vi "test Check Main Properties Changes.vi"(8 "error in":errorcluster, 11 "TestCase in":refnum<class "AIM ARINC 664 EncodeDecode.lvclass">) -> (0 "error out":errorcluster, 3 "TestCase out":refnum<class "AIM ARINC 664 EncodeDecode.lvclass">)   [LabVIEW 2020, in "AIM ARINC 664 EncodeDecode.lvclass"]
uses:
  AIM ARINC 664 EncodeDecode.lvclass
  C:/Program Files (x86)/National Instruments/LabVIEW 2020/vi.lib/NI/VeriStand Custom Device Testing Tools/VeriStandScriptingTestCase/VeriStandScriptingTestCase.lvclass
  Import/_typedefs/session_tx_generic.ctl
  Import/_typedefs/tx_generic_setup.ctl
  Import/_typedefs/frame_tx_generic.ctl
  Import/_typedefs/frame_tx_generic_seqNumberInit.ctl
  Import/_typedefs/frame_tx_generic_seqNumberOffset.ctl
  Import/_typedefs/frame_parameter.ctl
  Import/_typedefs/frame_parameter_definition.ctl
  <vilib>/NI/NI VeriStand Encoding and Decoding/Encoding.ctl
  Import/_typedefs/session_rx_monitor.ctl
  Import/_typedefs/board_setup.ctl
  <vilib>/NI/VeriStand Custom Device Testing Tools/VeriStandScriptingTestCase/VeriStandScriptingTestCase.lvclass/VeriStandScriptingTestCase.ctl
  <vilib>/NI/VeriStand Custom Device Testing Tools/VeriStandScriptingTestCase/Read Target.vi
  NationalInstruments.VeriStand.SystemDefinitionAPI
  <vilib>/addons/_JKI Toolkits/VI Tester/TestCase.llb/TestCase.lvclass
  Scripting/AIM ARINC 664 Scripting.lvlib
  Import/AIM ARINC 664 Import.lvlib
  <vilib>/NI/NI VeriStand Encoding and Decoding/Encoding and Decoding.lvlib
  C:/Program Files (x86)/National Instruments/LabVIEW 2020/vi.lib/addons/_JKI Toolkits/VI Tester/TestCase.llb/TestCase.lvclass
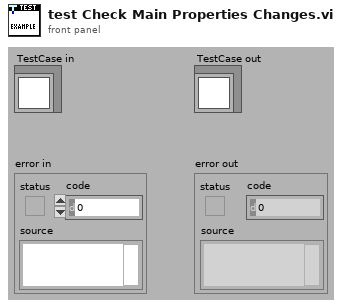
[diagram p1: front panel]
types:
  T1 = typedef "AIM ARINC 664 Import.lvlib/session_rx_monitor.ctl" = cluster{"DefaultCronoMode":u32, "GlbMonBufferSizeIn":u32, "CaptureMode":u32, "MaxFileSizeMB":u32, "Strobe":u32, "TriggerPosition":u32}
  T2 = typedef "AIM ARINC 664 Import.lvlib/session_tx_generic.ctl" = cluster{"tx_generic_setup":T3, "Frame Headers":T4[]}
  T3 = typedef "AIM ARINC 664 Import.lvlib/tx_generic_setup.ctl" = cluster{"QueueSizeIn":u32, "Count":i32, "StartMode":i32}
  T4 = typedef "AIM ARINC 664 Import.lvlib/frame_tx_generic.ctl" = cluster{"FrameID":string, "PayloadID":string, "Frame header":cluster{"FrameStartMode":i32, "InterFrameGap":i32, "PacketGroupWaitTime":i32, "NetSelect":u32, "PayloadBufferMode":i32, "PayloadGenerationMode":i32, "PhysErrorInjection":i32, "PreambleCount":i32, "SequenceNumberInit":T5, "SequenceNumberOffset":T6, "Skew":i32}, "Parameters":T7[]}
  T5 = typedef "AIM ARINC 664 Import.lvlib/frame_tx_generic_seqNumberInit.ctl" = i32
  T6 = typedef "AIM ARINC 664 Import.lvlib/frame_tx_generic_seqNumberOffset.ctl" = i32
  T7 = typedef "AIM ARINC 664 Import.lvlib/frame_parameter.ctl" = cluster{"name":string, "default value":dbl, "unit":string, "Parameter":T8}
  T8 = typedef "AIM ARINC 664 Import.lvlib/frame_parameter_definition.ctl" = cluster{"start index":i32, "size":i32, "encoding":T9, "signed":bool, "scale multiplier":dbl, "scale offset":dbl}
  T9 = typedef "Encoding and Decoding.lvlib/Encoding.ctl" = enum16{"BNR", "BCD", "Discrete"}
  T10 = typedef "AIM ARINC 664 Import.lvlib/board_setup.ctl" = cluster{"boardId":u32, "portSpeed":u32, "portConfig":u32}
  T11 = typedef "Custom Device API.lvlib/Custom Device Item Ref.ctl" = u64
  T12 = typedef "AIM ARINC 664 Import.lvlib/port_setup.ctl" = cluster{"port Id":u32, "redundant":bool}
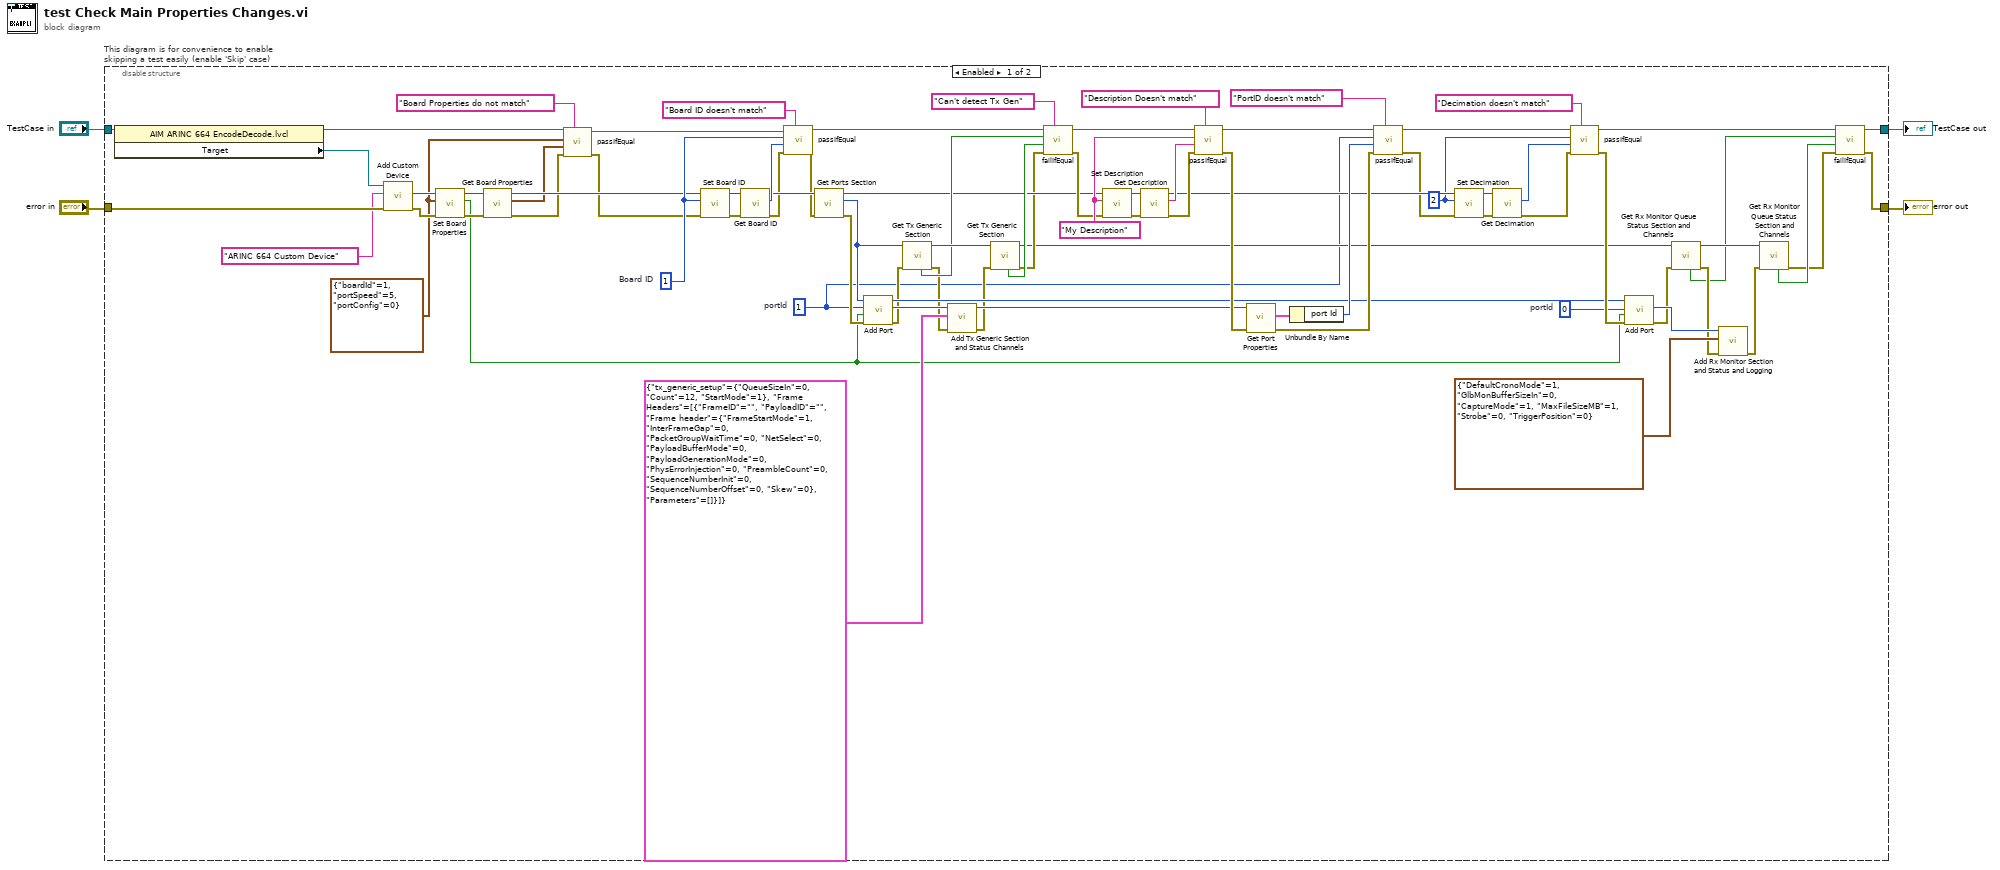
[diagram p0: block diagram]
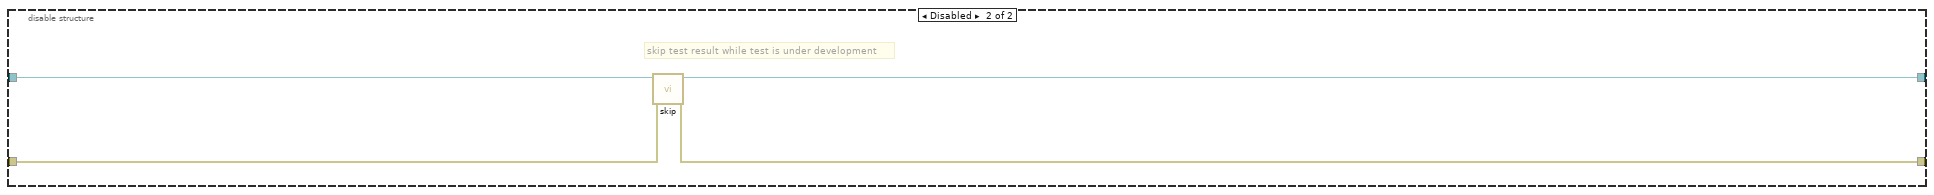
[diagram p2: hidden frame]
diagram:
  n1 = disable-structure "This diagram is for convenience to enable skipping a test easily (enable 'Skip' case)" shown="Enabled" {
    disable-tunnel: "TestCase in" -> [w83 w88]
    disable-tunnel: [w25 w86] -> w1
    disable-tunnel: [w21 w87] -> w3
    disable-tunnel: "error in" -> [w84 w85]
    frame Enabled {
      w11 = T10 {"boardId"=1, "portSpeed"=5, "portConfig"=0} ("board setup")
      w19 = u32 0  # portId
      w20 = u32 1  # portId
      w58 = 2 ("decimation")
      w76 = "My Description" ("description")
      w68 = 1  # Board ID
      n2 = property class="AIM ARINC 664 EncodeDecode.lvcl"(reference=w83) -> (reference out=w10:refnum<class "AIM ARINC 664 EncodeDecode.lvclass">, "Target"=w82:refnum<k24>)  [unwired: 1 in, 1 out]
      n3 = call "Add Custom Device.vi"("error in"=w84, "name"="ARINC 664 Custom Device", "target in"=w82) -> ("error out"=w15:errorcluster, "custom device"=w17:T11)  [unwired: 6 in, 1 out]
      n4 = call "Set Board Properties.vi"("error in"=w15, "board setup"=w11, "custom device ref in"=w17) -> ("error out"=w14:errorcluster, "redundant?"=w13:bool, "custom device ref out"=w16:T11)  [unwired: 6 in]
      n5 = call "Get Board Properties.vi"("error in"=w14, "custom device ref"=w16) -> ("error out"=w8:errorcluster, "board properties out"=w5:T10, "custom device ref out"=w12:T11)  [unwired: 7 in]
      n6 = call-dynamic "passIfEqual.vi"("custom report message (\"\")"="Board Properties do not match" ("custom report message (\"\")"), "error in (no error)"=w8, "y"=w5, "x"=w11, "TestCase in"=w10) -> ("error out"=w7:errorcluster, "TestCase out"=w9:refnum<class "AIM ARINC 664 EncodeDecode.lvclass">)  [unwired: 5 in]
      n7 = call "Set Board ID.vi"("error in"=w7, "Board ID"=w68, "custom device ref"=w12) -> ("error out"=w46:errorcluster, "custom device ref out"=w47:T11)  [unwired: 7 in]
      n8 = call "Get Board ID.vi"("error in"=w46, "custom device ref"=w47) -> ("error out"=w44:errorcluster, "Board ID"=w69:i32, "custom device ref out"=w45:T11)  [unwired: 7 in]
      n9 = call-dynamic "passIfEqual.vi"("custom report message (\"\")"="Board ID doesn't match" ("description"), "error in (no error)"=w44, "y"=w69, "x"=w68, "TestCase in"=w9) -> ("error out"=w18:errorcluster, "TestCase out"=w43:refnum<class "AIM ARINC 664 EncodeDecode.lvclass">)  [unwired: 5 in]
      n10 = call "Get Ports Section.vi"("error in"=w18, "custom device ref"=w45) -> ("error out"=w80:errorcluster, "ports ref out"=w48:T11, "custom device ref out"=w36:T11)  [unwired: 6 in, 1 out]
      n11 = call "Add Port.vi"("error in"=w80, "redundant ?"=w13, "port Id"=w20, "ports ref"=w48) -> ("error out"=w49:errorcluster, "port ref out"=w64:T11, "ports ref out"=w53:T11)  [unwired: 5 in]
      n12 = call "Get Tx Generic Section.vi"("error in"=w49, "Parent section Ref in"=w48) -> ("error out"=w34:errorcluster, "Parent section Ref out"=w41:T11, "found?"=w40:bool)  [unwired: 6 in, 1 out]
      n13 = call "Add Tx Generic Section and Status Channels.vi"("error in"=w34, "Tx generic configuration"=T2 {"tx_generic_setup"={"QueueSizeIn"=0, "Count"=12, "StartMode"=1}, "Frame Headers"=[{"FrameID"="", "PayloadID"="", "Frame header"={"FrameStartMode"=1, "InterFrameGap"=0, "PacketGroupWaitTime"=0, "NetSelect"=0, "PayloadBufferMode"=0, "PayloadGenerationMode"=0, "PhysErrorInjection"=0, "PreambleCount"=0, "SequenceNumberInit"=0, "SequenceNumberOffset"=0, "Skew"=0}, "Parameters"=[]}]}, "port ref"=w64) -> ("error out"=w33:errorcluster, "port ref out"=w50:T11)  [unwired: 7 in]
      n14 = call "Get Tx Generic Section.vi"("error in"=w33, "Parent section Ref in"=w41) -> ("error out"=w35:errorcluster, "Parent section Ref out"=w31:T11, "found?"=w39:bool)  [unwired: 6 in, 1 out]
      n15 = call-dynamic "failIfEqual.vi"("custom report message (\"\")"="Can't detect Tx Gen" ("custom report message (\"\")"), "error in (no error)"=w35, "y"=w39, "x"=w40, "TestCase in"=w43) -> ("error out"=w38:errorcluster, "TestCase out"=w42:refnum<class "AIM ARINC 664 EncodeDecode.lvclass">)  [unwired: 5 in]
      n16 = call "Set Description.vi"("error in"=w38, "description"=w76, "custom device ref"=w36) -> ("error out"=w77:errorcluster, "custom device ref out"=w78:T11)  [unwired: 7 in]
      n17 = call "Get Description.vi"("error in"=w77, "custom device ref"=w78) -> ("error out"=w75:errorcluster, "description"=w67:string, "custom device ref out"=w62:T11)  [unwired: 7 in]
      n18 = call-dynamic "passIfEqual.vi"("custom report message (\"\")"="Description Doesn't match" ("custom report message (\"\")"), "error in (no error)"=w75, "y"=w67, "x"=w76, "TestCase in"=w42) -> ("error out"=w74:errorcluster, "TestCase out"=w72:refnum<class "AIM ARINC 664 EncodeDecode.lvclass">)  [unwired: 5 in]
      n19 = call "Get Port Properties.vi"("error in"=w74, "custom device ref"=w50) -> ("error out"=w70:errorcluster, "port properties out"=w73:T12)  [unwired: 7 in, 1 out]
      n20 = Unbundle By Name(w73) -> ("port Id"=w71:u32)
      n21 = call-dynamic "passIfEqual.vi"("custom report message (\"\")"="PortID doesn't match" ("description"), "error in (no error)"=w70, "y"=w71, "x"=w20, "TestCase in"=w72) -> ("error out"=w61:errorcluster, "TestCase out"=w55:refnum<class "AIM ARINC 664 EncodeDecode.lvclass">)  [unwired: 5 in]
      n22 = call "Set Decimation.vi"("error in"=w61, "decimation"=w58, "custom device ref"=w62) -> ("error out"=w60:errorcluster, "custom device ref out"=w57:T11)  [unwired: 7 in]
      n23 = call "Get Decimation.vi"("error in"=w60, "custom device ref"=w57) -> ("error out"=w59:errorcluster, "decimation"=w56:i32)  [unwired: 7 in, 1 out]
      n24 = call-dynamic "passIfEqual.vi"("custom report message (\"\")"="Decimation doesn't match" ("description"), "error in (no error)"=w59, "y"=w56, "x"=w58, "TestCase in"=w55) -> ("error out"=w54:errorcluster, "TestCase out"=w26:refnum<class "AIM ARINC 664 EncodeDecode.lvclass">)  [unwired: 5 in]
      n25 = call "Add Port.vi"("error in"=w54, "redundant ?"=w13, "port Id"=w19, "ports ref"=w53) -> ("error out"=w32:errorcluster, "port ref out"=w52:T11)  [unwired: 5 in, 1 out]
      n26 = call "Get Rx Monitor Queue Status Section and Channels.vi"("error in"=w32, "custom device ref in"=w31) -> ("error out"=w29:errorcluster, "custom device ref out"=w27:T11, "found?"=w24:bool)  [unwired: 5 in, 2 out]
      n27 = call "Add Rx Monitor Section and Status and Logging.vi"("error in"=w29, "session_rx_monitor"=T1 {"DefaultCronoMode"=1, "GlbMonBufferSizeIn"=0, "CaptureMode"=1, "MaxFileSizeMB"=1, "Strobe"=0, "TriggerPosition"=0}, "port ref"=w52) -> ("error out"=w28:errorcluster)  [unwired: 7 in, 1 out]
      n28 = call "Get Rx Monitor Queue Status Section and Channels.vi"("error in"=w28, "custom device ref in"=w27) -> ("error out"=w22:errorcluster, "found?"=w23:bool)  [unwired: 5 in, 3 out]
      n29 = call-dynamic "failIfEqual.vi"("error in (no error)"=w22, "y"=w23, "x"=w24, "TestCase in"=w26) -> ("error out"=w21:errorcluster, "TestCase out"=w25:refnum<class "AIM ARINC 664 EncodeDecode.lvclass">)  [unwired: 6 in]
    }
    frame Disabled {
      # "skip test result while test is under development"
      n30 = call <vilib>:"skip.vi"("error in (no error)"=w85, "TestCase in"=w88) -> ("error out"=w87:errorcluster, "TestCase out"=w86:refnum<class "AIM ARINC 664 EncodeDecode.lvclass">)  [unwired: 8 in]
    }
  }
  "error out" <- w3
  "TestCase out" <- w1
